vi "ElectdClear.vi"(11 "Electd in":refnum<vi>) -> (3 "Electd out":refnum<vi>)   [LabVIEW 2012, in "StimulCtrls.lvlib"]
uses:
  StimulCtrls.lvlib
  ElectdPanel.ctl
  ElectdTerminal.ctl
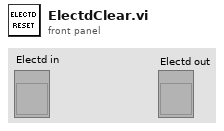
[diagram p1: front panel]
types:
  T1 = enum8{"Enabled", "Disabled", "Disabled and Grayed Out"}
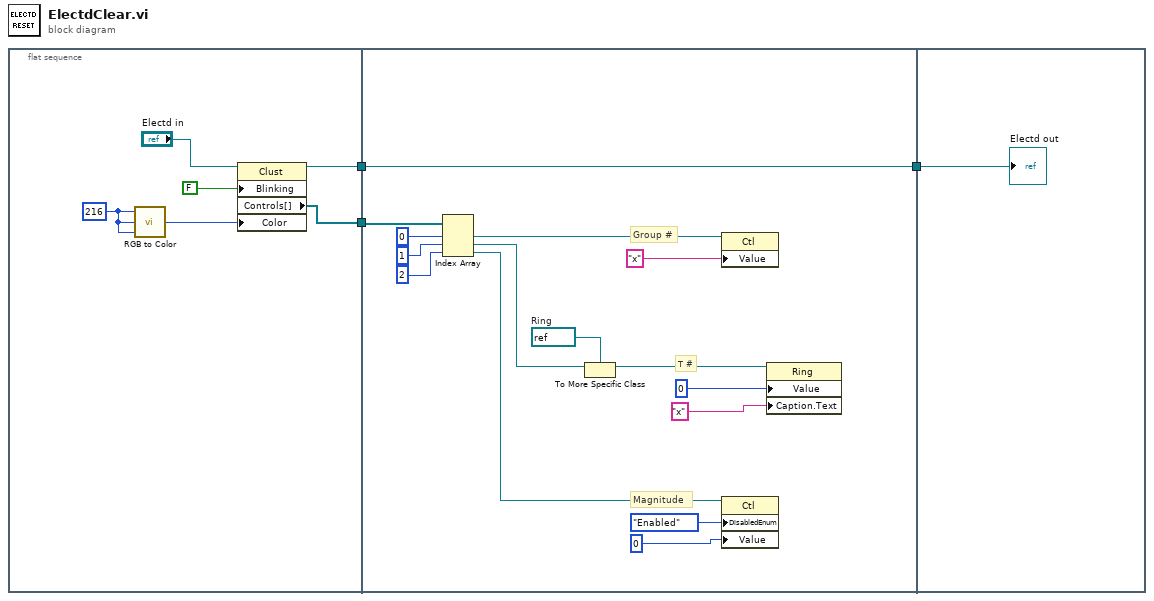
[diagram p0: block diagram]
diagram:
  n1 = flat-sequence {
    tunnel: [w7] -> w3
    tunnel: [w6] -> w2
    tunnel: w3 -> [w13]
    tunnel: w2 -> [w12]
    tunnel: [w12] -> w1
    tunnel: w1 -> [w25]
    frame #0 {
      w5 = u8 216 ("R")
      n2 = call <vilib>:"RGB to Color.vi"("B"=w5, "G"=w5, "R"=w5) -> ("Color"=w4:u32)
      n3 = property class="Clust"(reference="Electd in", "Blinking"=FALSE, "Color"=w4) -> (reference out=w6:refnum<vi>, "Controls[]"=w7:refnum<vi>[])  [unwired: 1 in, 1 out]
    }
    frame #1 {
      w10 = refnum<vi> refnum  # Ring
      # "Group #"
      # "Magnitude"
      # "T #"
      n4 = Index Array(array=w13, index #1=0 ("index"), index #2=1 ("index"), index #3=2 ("index")) -> (element #1=w14:refnum<vi>, element #2=w15:refnum<vi>, element #3=w16:refnum<vi>)
      n5 = To More Specific Class(target class=w10, reference=w15) -> (specific class reference=w11:refnum<vi>)  [unwired: 1 in, 1 out]
      n6 = property class="Ctl"(reference=w14, "Value"="x") -> ()  [unwired: 1 in, 2 out]
      n7 = property class="Ctl"(reference=w16, "DisabledEnum"=T1."Enabled" ("Disabled"), "Value"=0) -> ()  [unwired: 1 in, 2 out]
      n8 = property class="Ring"(reference=w11, "Value"=0, "Caption.Text"="x") -> ()  [unwired: 1 in, 2 out]
    }
    frame #2 {
      "Electd out" <- w25
    }
  }
